vi "Example.vi"() -> ()   [LabVIEW 2023, in "Freetype Drawer.lvlib"]
uses:
  Freetype Drawer.lvlib
  Glyph Slot Rec.ctl
  FT Metrics RAW.ctl
  FT Bitmap.ctl
  Face.ctl
  FT Metrics.ctl
  Bitmap Glyph.ctl
  Glyph Rec.ctl
  Font Glyph Drawer Interface/Font Glyph Drawer Interface.lvlib
panel:
  out "Box 2":T1
  out "Box":T1
  out "Bitmap Glyph Rec":T2
  out "bitmap":T4
  out "metrics":T5
  out "2D Picture":picture
  out "index":u32
  out "library":i64
  out "glyph ref out":i64
  out "Face":T6
  out "out":T7
  out "Family Name":string
  out "error out":errorcluster
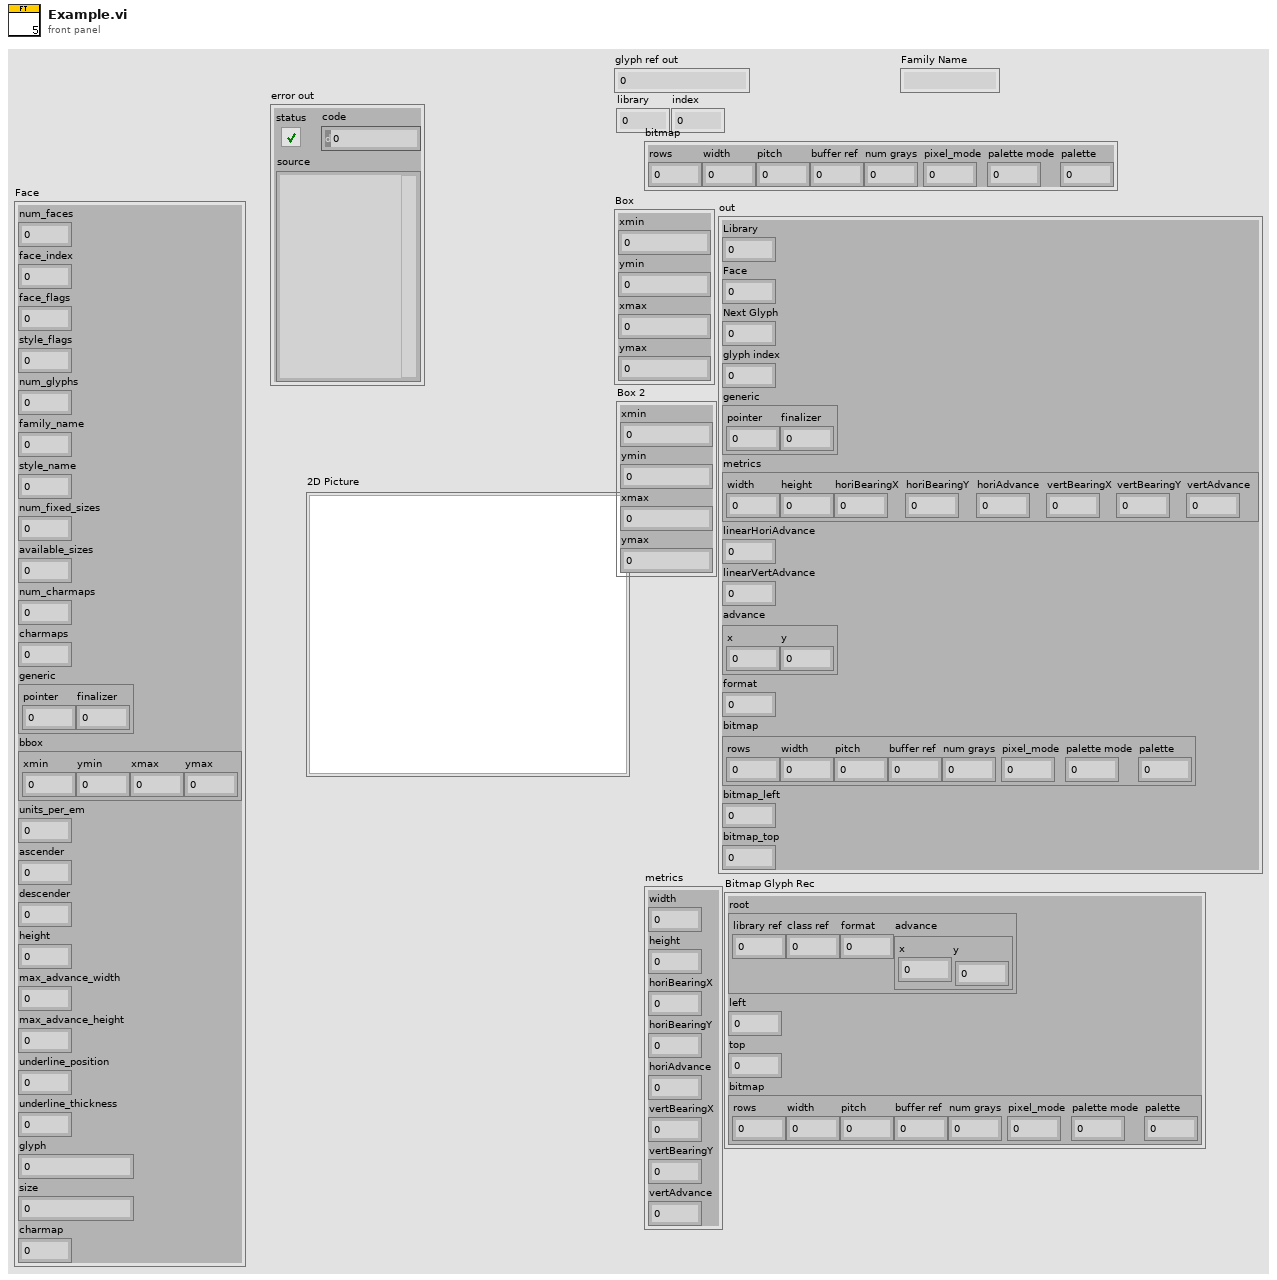
[diagram p1: front panel]
types:
  T1 = cluster{"xmin":dbl, "ymin":dbl, "xmax":dbl, "ymax":dbl}
  T2 = typedef "Freetype Drawer.lvlib/Bitmap Glyph.ctl" = cluster{"root":T3, "left":i32, "top":i32, "bitmap":T4}
  T3 = typedef "Freetype Drawer.lvlib/Glyph Rec.ctl" = cluster{"library ref":i64, "class ref":i64, "format":i32, "advance":cluster{"x":i32, "y":i32}}
  T4 = typedef "Freetype Drawer.lvlib/FT Bitmap.ctl" = cluster{"rows":u32, "width":u32, "pitch":i32, "buffer ref":i64, "num grays":i16, "pixel_mode":u8, "palette mode":u8, "palette":i64}
  T5 = typedef "Freetype Drawer.lvlib/FT Metrics.ctl" = cluster{"width":sgl, "height":sgl, "horiBearingX":sgl, "horiBearingY":sgl, "horiAdvance":sgl, "vertBearingX":sgl, "vertBearingY":sgl, "vertAdvance":sgl}
  T6 = typedef "Freetype Drawer.lvlib/Face.ctl" = cluster{"num_faces":i32, "face_index":i32, "face_flags":i32, "style_flags":i32, "num_glyphs":i32, "family_name":i64, "style_name":i64, "num_fixed_sizes":i32, "available_sizes":i64, "num_charmaps":i32, "charmaps":i64, "generic":cluster{"pointer":i64, "finalizer":i64}, "bbox":cluster{"xmin":i32, "ymin":i32, "xmax":i32, "ymax":i32}, "units_per_em":u16, "ascender":i16, "descender":i16, "height":i16, "max_advance_width":i16, "max_advance_height":i16, "underline_position":i16, "underline_thickness":i16, "glyph":i64, "size":i64, "charmap":i64}
  T7 = typedef "Freetype Drawer.lvlib/Glyph Slot Rec.ctl" = cluster{"Library":i64, "Face":i64, "Next Glyph":i64, "glyph index":u32, "generic":cluster{"pointer":i64, "finalizer":i64}, "metrics":T8, "linearHoriAdvance":i32, "linearVertAdvance":i32, "advance":cluster{"x":i32, "y":i32}, "format":i32, "bitmap":T4, "bitmap_left":i32, "bitmap_top":i32}
  T8 = typedef "Freetype Drawer.lvlib/FT Metrics RAW.ctl" = cluster{"width":i32, "height":i32, "horiBearingX":i32, "horiBearingY":i32, "horiAdvance":i32, "vertBearingX":i32, "vertBearingY":i32, "vertAdvance":i32}
  T9 = typedef "NI_Matrix.lvlib/RealMatrix.ctl" = dbl[][]
  T10 = typedef "Freetype Drawer.lvlib/Outline Glyph Rec.ctl" = cluster{"root":T3, "Outline":cluster{"n_contours":i16, "n_points":i16, "points ref":i64, "tags ref":i64, "contours ref":i64, "flags":i32}}
  T11 = cluster{"xmin":sgl, "ymin":sgl, "xmax":sgl, "ymax":sgl}
  T12 = typedef "imagedata.ctl" = cluster{"image type":i32, "image depth":i32, "image":u8[], "mask":u8[], "colors":u32[], "Rectangle":cluster{"left":i16, "top":i16, "right":i16, "bottom":i16}}
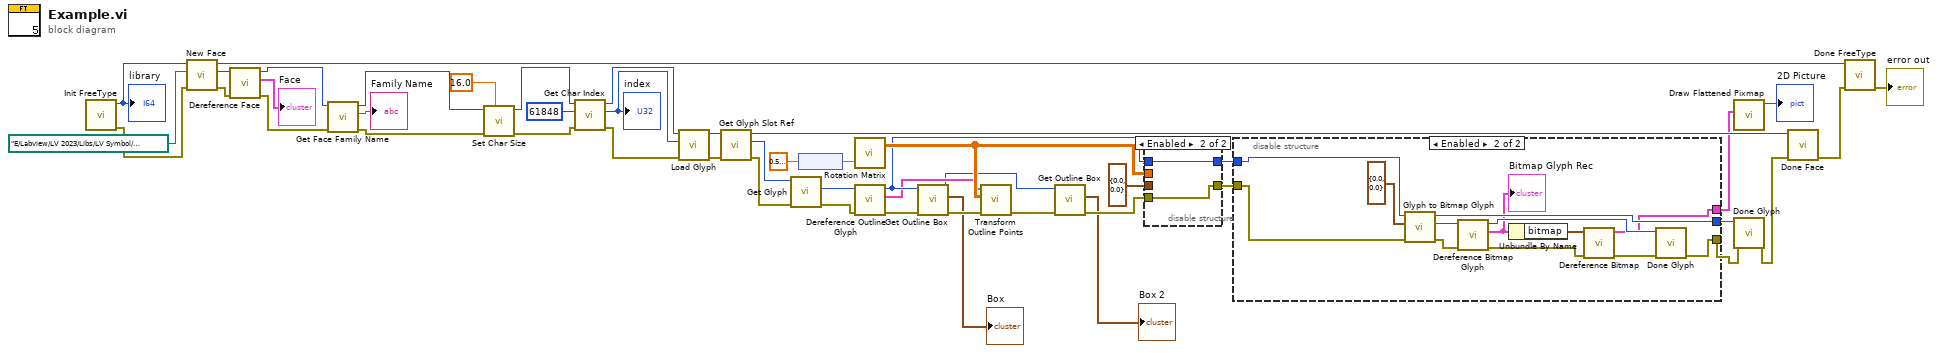
[diagram p0: block diagram]
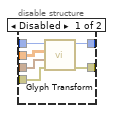
[diagram p2: hidden frame]
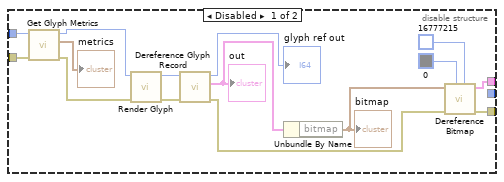
[diagram p3: hidden frame]
diagram:
  n1 = call "Init FreeType.vi"() -> ("error out"=w47:errorcluster, "library"=w31:i64)  [unwired: 10 in]
  "library" <- w31
  n2 = call "New Face.vi"("error in (no error)"=w47, "Path"=path "E:/Labview/LV 2023/Libs/LV Symbol/LV-Awesome/fonts/elusiveicons-webfont.ttf", "library in"=w31) -> ("error out"=w48:errorcluster, "face out"=w38:i64, "library out"=w45:i64)  [unwired: 6 in]
  n3 = call "Dereference Face.vi"("error in (no error)"=w48, "face in"=w38) -> ("error out"=w39:errorcluster, "Face"=→"Face":T6, "face out"=w37:i64)  [unwired: 7 in]
  n4 = call "Get Face Family Name.vi"("error in (no error)"=w39, "face in"=w37) -> ("error out"=w42:errorcluster, "Family Name"=→"Family Name":string, "face out"=w23:i64)  [unwired: 7 in]
  n5 = call "Set Char Size.vi"("height"=sgl 16.0, "error in (no error)"=w42, "face in"=w23) -> ("error out"=w33:errorcluster, "face out"=w29:i64)  [unwired: 7 in]
  n6 = call "Get Char Index.vi"("error in (no error)"=w33, "charcode"=u32 61848 ("glyph_index"), "face"=w29) -> ("error out"=w30:errorcluster, "index"=w26:u32, "face out"=w28:i64)  [unwired: 6 in]
  "index" <- w26
  n7 = call "Load Glyph.vi"("error in (no error)"=w30, "glyph_index"=w26, "face in"=w28) -> ("error out"=w35:errorcluster, "face out"=w34:i64)  [unwired: 7 in]
  n8 = call "Get Glyph Slot Ref.vi"("error in (no error)"=w35, "face in"=w34) -> ("error out"=w17:errorcluster, "glyph slot ref"=w18:i64, "face out"=w40:i64)  [unwired: 7 in]
  n9 = call "Get Glyph.vi"("error in (no error)"=w17, "glyph slot ref in"=w18) -> ("error out"=w20:errorcluster, "glyph ref out"=w9:i64)  [unwired: 7 in, 1 out]
  n10 = node(dbl[unit] 0.5235987755982988 ("Rotation rad")) -> (w21:dbl)
  n11 = call "Rotation Matrix.vi"("Rotation rad"=w21) -> ("Matrix Out"=w8:T9)  [unwired: 2 in]
  n12 = call "Dereference Outline Glyph.vi"("error in (no error)"=w20, "glyph ref in"=w9) -> ("error out"=w10:errorcluster, "Outline Glyph Rec"=w2:T10, "glyph ref out"=w3:i64)  [unwired: 7 in]
  n13 = call "Get Outline Box.vi"("error in (no error)"=w10, "contour glyph ref"=w3) -> ("error out"=w7:errorcluster, "Box"=→"Box":T11, "contour glyph ref dup"=w1:i64)  [unwired: 6 in, 1 out]
  n14 = call "Transform Outline Points.vi"("error in (no error)"=w7, "2xN Matrix"=w8, "Outline Glyph Rec"=w2) -> ("error out"=w11:errorcluster)  [unwired: 7 in, 1 out]
  n15 = call "Get Outline Box.vi"("error in (no error)"=w11, "contour glyph ref"=w1) -> ("error out"=w5:errorcluster, "Box"=→"Box 2":T11)  [unwired: 6 in, 2 out]
  n16 = disable-structure shown="Enabled" {
    disable-tunnel: cluster{"x":sgl, "y":sgl} {"x"=0.0, "y"=0.0} ("Offset") -> [w54 _]
    disable-tunnel: [w53 w55] -> w16
    disable-tunnel: [w52 w56] -> w13
    disable-tunnel: w5 -> [w51 w55]
    disable-tunnel: w3 -> [w50 w56]
    disable-tunnel: w8 -> [w49 _]
    frame Disabled {
      n17 = call "Glyph Transform.vi"("error in (no error)"=w51, "Offset"=w54, "Matrix"=w49, "glyph ref"=w50) -> ("error out"=w53:errorcluster, "glyph ref"=w52:i64)  [unwired: 6 in]
    }
    frame Enabled {
    }
  }
  n18 = disable-structure shown="Enabled" {
    disable-tunnel: [w68 w80] -> w15
    disable-tunnel: [w67 w74] -> w24
    disable-tunnel: w13 -> [w59 w83]
    disable-tunnel: w16 -> [w58 w84]
    disable-tunnel: [_ w82] -> w12
    frame Disabled {
      n19 = call "Get Glyph Metrics.vi"("error in (no error)"=w58, "glyph ref in"=w59) -> ("error out"=w66:errorcluster, "metrics"=→"metrics":T5, "glyph ref out"=w65:i64)  [unwired: 7 in]
      n20 = call "Render Glyph.vi"("error in (no error)"=w66, "glyph slot"=w65) -> ("error out"=w71:errorcluster, "glyph slot 2"=w70:i64)  [unwired: 8 in]
      n21 = call "Dereference Glyph Record.vi"("error in (no error)"=w71, "glyph ref in"=w70) -> ("error out"=w57:errorcluster, "out"=w69:T7, "glyph ref out"=→"glyph ref out":i64)  [unwired: 7 in]
      "out" <- w69
      n22 = Unbundle By Name(w69) -> ("bitmap"=w63:T4)
      "bitmap" <- w63
      n23 = call "Dereference Bitmap.vi"("Back"=u32 16777215, "Front"=u32 0, "error in (no error)"=w57, "bitmap"=w63) -> ("error out"=w68:errorcluster, "image data"=w67:T12)  [unwired: 6 in]
    }
    frame Enabled {
      n24 = call "Glyph to Bitmap Glyph.vi"("error in (no error)"=w84, "Offset"=cluster{"x":sgl, "y":sgl} {"x"=0.0, "y"=0.0}, "glyph ref in"=w83) -> ("error out"=w81:errorcluster, "bitmap glyph ref out"=w79:i64, "glyph ref out"=w82:i64)  [unwired: 6 in]
      n25 = call "Dereference Bitmap Glyph.vi"("error in (no error)"=w81, "glyph ref in"=w79) -> ("error out"=w77:errorcluster, "Bitmap Glyph Rec"=w72:T2, "glyph ref out"=w78:i64)  [unwired: 7 in]
      "Bitmap Glyph Rec" <- w72
      n26 = Unbundle By Name(w72) -> ("bitmap"=w75:T4)
      n27 = call "Dereference Bitmap.vi"("error in (no error)"=w77, "bitmap"=w75) -> ("error out"=w76:errorcluster, "image data"=w74:T12)  [unwired: 8 in]
      n28 = call "Done Glyph.vi"("error in (no error)"=w76, "glyph ref in"=w78) -> ("error out"=w80:errorcluster)  [unwired: 9 in]
    }
  }
  n29 = call <vilib>:"Draw Flattened Pixmap.vi"("image data"=w24) -> ("new picture"=→"2D Picture":picture)  [unwired: 8 in]
  n30 = call "Done Glyph.vi"("error in (no error)"=w15, "glyph ref in"=w12) -> ("error out"=w14:errorcluster)  [unwired: 9 in]
  n31 = call "Done Face.vi"("error in (no error)"=w14, "face in"=w40) -> ("error out"=w44:errorcluster)  [unwired: 9 in]
  n32 = call "Done FreeType.vi"("error in (no error)"=w44, "library in"=w45) -> ("error out"=→"error out":errorcluster)  [unwired: 9 in]
